vi "RTS Save OpenClose Ref.vi"(6 "Custom Saved Titles":string[][](array[string]), 7 "Save Status 8":bool, 8 "error in (no error)":errorcluster, 9 "Setup Info Station 8":string[][](array[string]), 10 "CSV File Location 8":path, 11 "Byte Stream File in":refnum<file>) -> (0 "error out":errorcluster, 2 "CSV File Location Output":path, 3 "Byte Stream File out":refnum<file>)   [LabVIEW 2016]
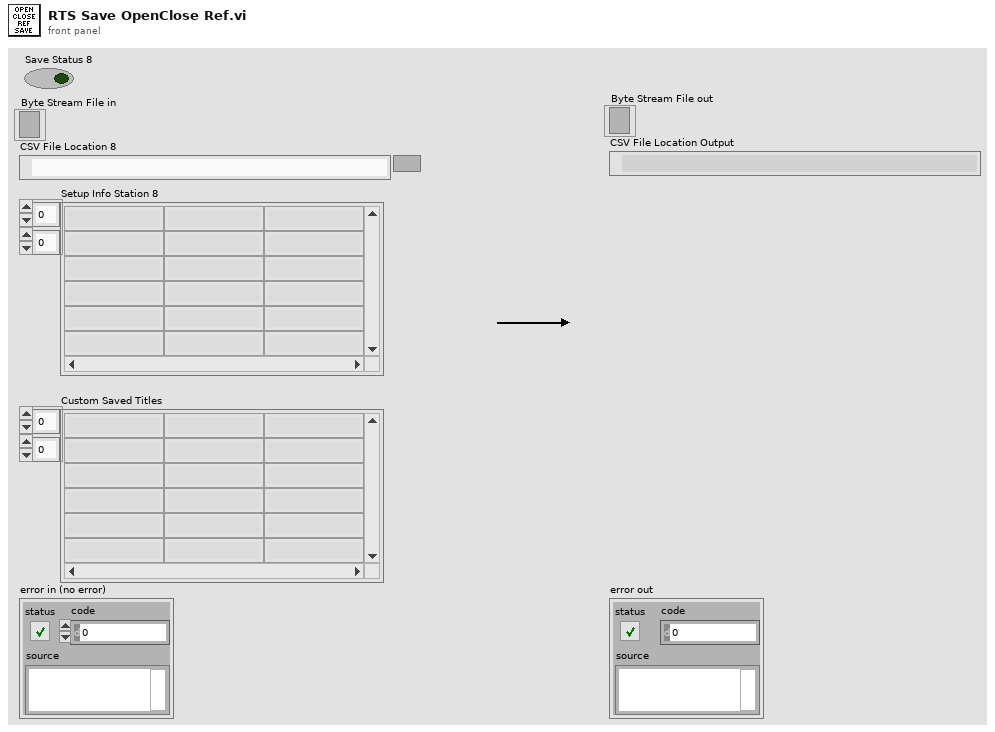
[diagram p1: front panel]
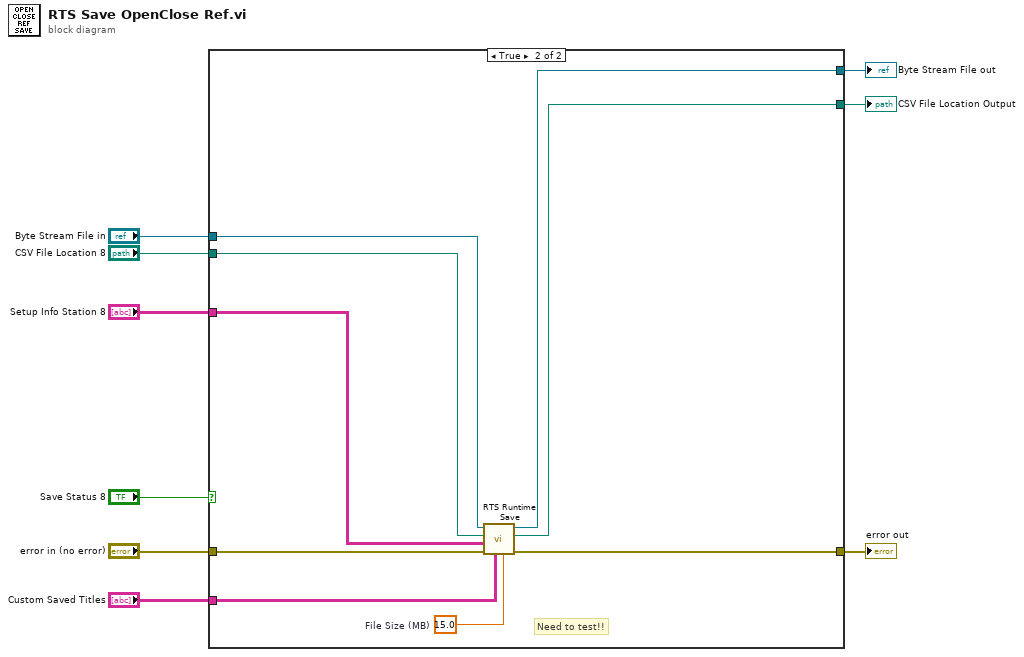
[diagram p0: block diagram]
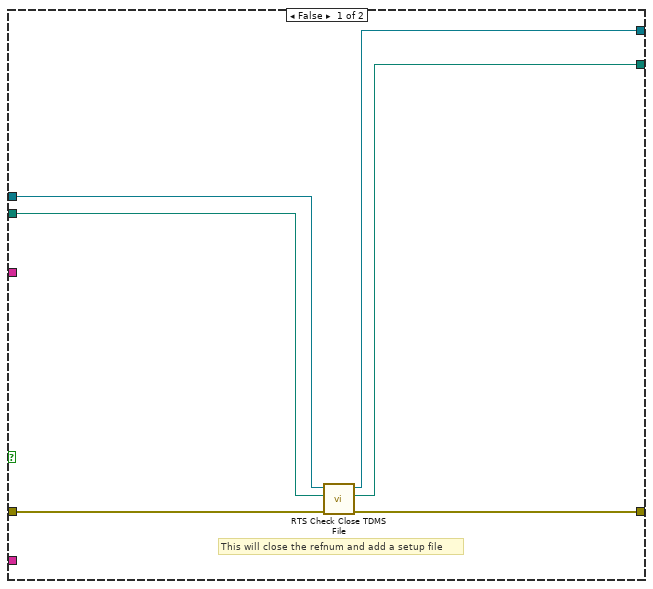
[diagram p2: hidden frame]
diagram:
  n1 = case shown="True" "Save Status 8" {
    tunnel: "error in (no error)" -> [w15 w24]
    tunnel: [w14 w19] -> w2
    tunnel: "CSV File Location 8" -> [w11 w20]
    tunnel: "Setup Info Station 8" -> [_ w23]
    tunnel: "Custom Saved Titles" -> [_ w18]
    tunnel: "Byte Stream File in" -> [w13 w21]
    tunnel: [w12 w22] -> w7
    tunnel: [w10 w17] -> w8
    frame False {
      # "This will close the refnum and add a setup file"
      n2 = call "RTS Check Close TDMS File.vi"("error in (no error)"=w15, "CSV File Location In"=w11, "Byte Stream In"=w13) -> ("error out"=w14:errorcluster, "CSV File Location Out"=w10:path, "Byte Stream Out"=w12:refnum<file>)  [unwired: 6 in]
    }
    frame True {
      w16 = 15.0  # File Size (MB)
      # "Need to test!!"
      n3 = call "RTS Runtime Save.vi"("File Size"=w16, "Custom Saved Titles"=w18, "error in (no error)"=w24, "Setup Info Station 8"=w23, "CSV File Location Input"=w20, "Byte Stream File in"=w21) -> ("error out"=w19:errorcluster, "CSV File Location Output"=w17:path, "Byte Stream File out"=w22:refnum<file>)  [unwired: 3 in]
    }
  }
  "CSV File Location Output" <- w8
  "Byte Stream File out" <- w7
  "error out" <- w2
